vi "Calibrate.vi"(0 "VISA resource name":refnum<visa-resource-name>, 5 "Calibration (0:All)":i32(ring) items=["All", "Level", "Local Leak Suppress", "Band"], 11 "error in (no error)":errorcluster) -> (4 "VISA resource name out":refnum<visa-resource-name>, 15 "error out":errorcluster)   [LabVIEW 2020, in "Anritsu Signal Analyzer Series.lvlib"]
doc: "Executes calibration."
uses:
  Anritsu Signal Analyzer Series.lvlib
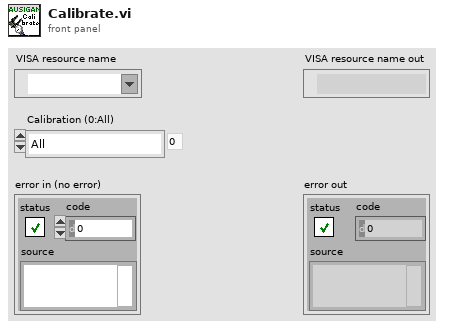
[diagram p1: front panel]
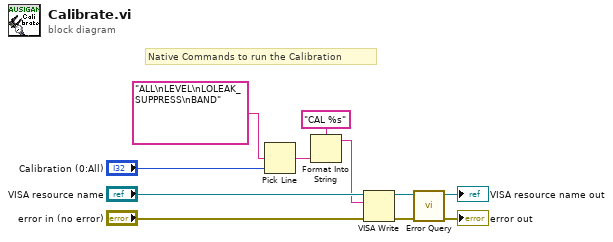
[diagram p0: block diagram]
diagram:
  # "Native Commands to run the Calibration"
  n1 = Pick Line(multi-line string="ALL\nLEVEL\nLOLEAK_SUPPRESS\nBAND" ("文字列"), line index="Calibration (0:All)") -> (output string=w3:string)  [unwired: 1 in]
  n2 = Format Into String(format string="CAL %s" ("形式文字列"), w3) -> (resulting string=w4:string)  [unwired: 2 in, 1 out]
  n3 = VISA Write(VISA resource name="VISA resource name", write buffer=w4, error in (no error)="error in (no error)") -> (VISA resource name out=w7:refnum<visa-resource-name>, error out=w6:errorcluster)  [unwired: 1 out]
  n4 = call "Error Query.vi"("error in (no error)"=w6, "VISA resource name"=w7) -> ("error out"=→"error out":errorcluster, "VISA resource name out"=→"VISA resource name out":refnum<visa-resource-name>)  [unwired: 6 in, 2 out]
